vi "ANAL_TimeSummer.vi"(9 "Target Set Points":i32[](array[numeric]), 10 "Software Gate":cluster{"Numeric":i32, "Numeric":i32}, 11 "Run Data Cluster":T2 {"Temperature B" scale=0.0..100.0; "Temperature A" scale=0.0..100.0}) -> (2 "Time Array":T1(array[cluster]))   [LabVIEW 2021]
uses:
  DAT_Cluster.ctl
  2ce880be-73f0-4406-b417-1ac9331a85e2.vi
  2ce880be-73f0-4406-b417-1ac9331a85e2.vi/d4db2432-cc9c-482c-8957-dac855435ef6.vi
  2ce880be-73f0-4406-b417-1ac9331a85e2.vi/86fbf154-bd7b-49a2-8ab2-a837b2a95f24.vi
  2ce880be-73f0-4406-b417-1ac9331a85e2.vi/3b95b01e-1ec2-4565-bcd9-7606a5281010.vi
  2ce880be-73f0-4406-b417-1ac9331a85e2.vi/96a08935-737a-44b2-979c-a81d56408f7e.vi
  2ce880be-73f0-4406-b417-1ac9331a85e2.vi/d4db2432-cc9c-482c-8957-dac855435ef6.vi/6eaecd13-6e48-4772-a921-b51ebdf84d88.vi
  2ce880be-73f0-4406-b417-1ac9331a85e2.vi/d4db2432-cc9c-482c-8957-dac855435ef6.vi/d2d5f2b7-06f4-47f6-971c-049c3fdbb653.vi
  2ce880be-73f0-4406-b417-1ac9331a85e2.vi/3b95b01e-1ec2-4565-bcd9-7606a5281010.vi/6eaecd13-6e48-4772-a921-b51ebdf84d88.vi
  2ce880be-73f0-4406-b417-1ac9331a85e2.vi/3b95b01e-1ec2-4565-bcd9-7606a5281010.vi/d2d5f2b7-06f4-47f6-971c-049c3fdbb653.vi
  2ce880be-73f0-4406-b417-1ac9331a85e2.vi/96a08935-737a-44b2-979c-a81d56408f7e.vi/6eaecd13-6e48-4772-a921-b51ebdf84d88.vi
  2ce880be-73f0-4406-b417-1ac9331a85e2.vi/96a08935-737a-44b2-979c-a81d56408f7e.vi/d2d5f2b7-06f4-47f6-971c-049c3fdbb653.vi
  <vilib>/Comparison/Less/Less Functor/Less Functor.lvclass
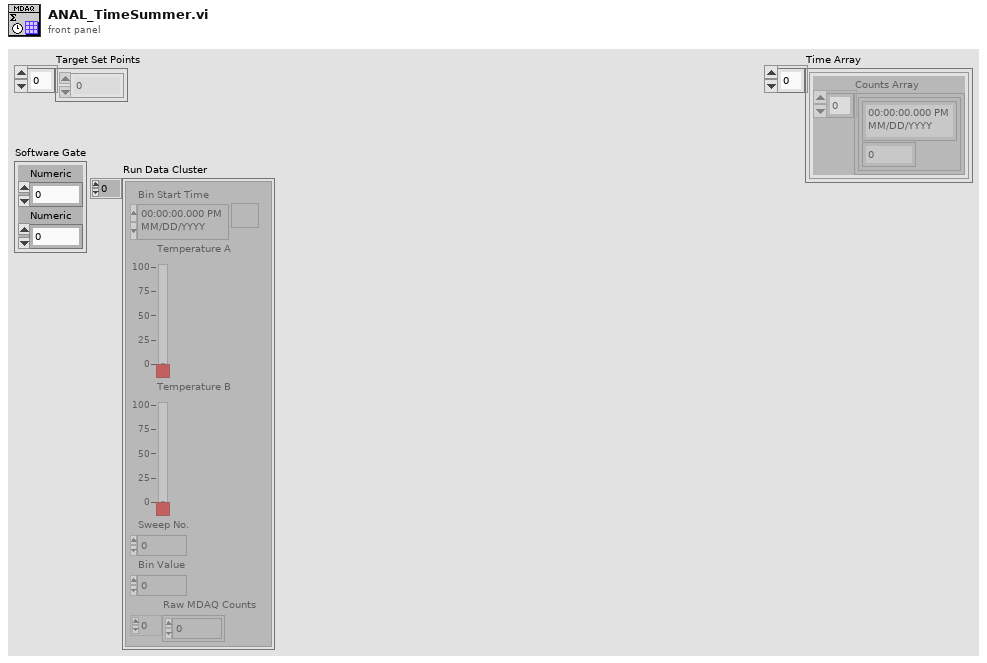
[diagram p1: front panel]
types:
  T1 = cluster{"Counts Array":cluster{timestamp, dbl}[]}[]
  T2 = typedef "DAT_Cluster.ctl" = cluster{"Bin Start Time":timestamp, "Temperature A":dbl, "Temperature B":dbl, "Sweep No.":i32, "Bin Value":i32, "Raw MDAQ Counts":i32[]}[]
  T3 = cluster{"Bin Start Time":timestamp, "Numeric":i32, "nearest index":i32}[]
  T4 = cluster{"Counts Array":cluster{timestamp, dbl}[]}
  T5 = cluster{"Bin Start Time":timestamp, "Numeric":i32, "nearest index":i32}
  T6 = cluster{"Bin Start Time":timestamp, "Numeric":i32}
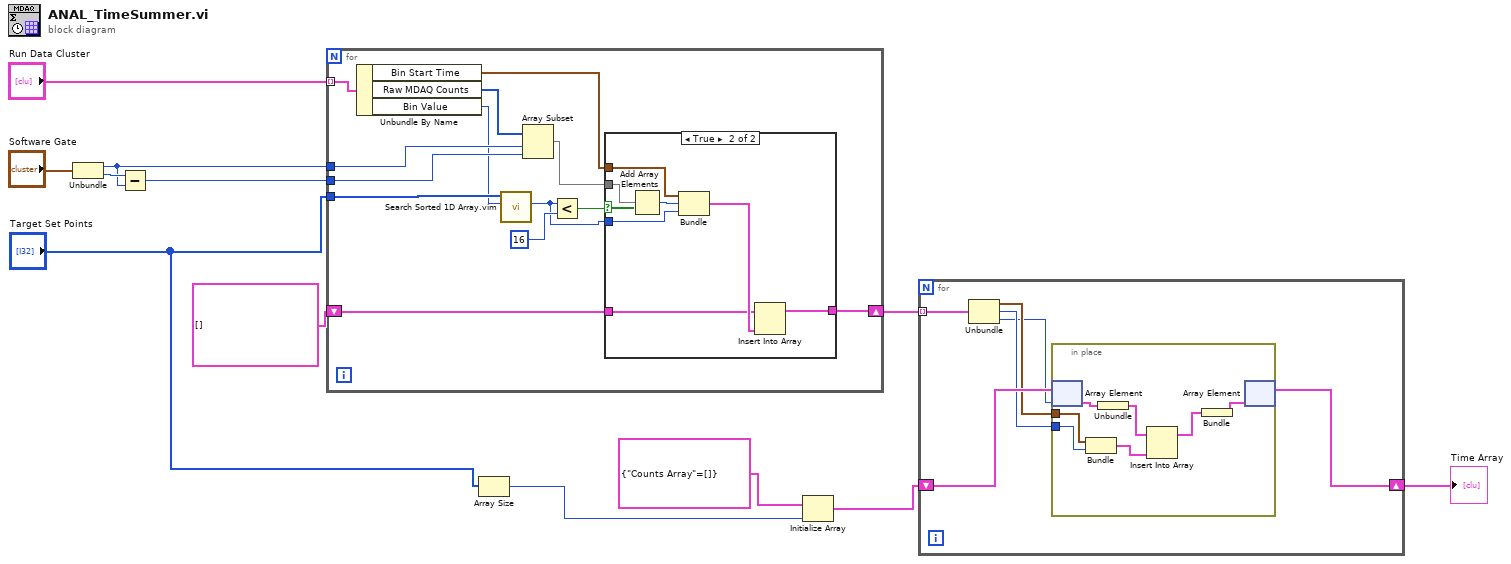
[diagram p0: block diagram]
diagram:
  n1 = Unbundle("Software Gate") -> ("Numeric"=w9:i32, "Numeric"=w10:i32)
  n2 = Subtract(x=w10, y=w9) -> (x-y=w8:i32)
  n3 = for {
    tunnel: "Run Data Cluster" -> [w25] mode=indexing
    tunnel: w9 -> [w23]
    tunnel: w8 -> [w22]
    tunnel: "Target Set Points" -> [w21]
    shift-right: [w14] -> w7
    shift-left: T3 [] ("array") -> [w15]
    n4 = Unbundle By Name(w25) -> ("Bin Start Time"=w18:timestamp, "Raw MDAQ Counts"=w24:i32[], "Bin Value"=w16:i32)
    n5 = call "Search Sorted 1D Array.vim"("element"=w16, "sorted 1D array"=w21) -> ("nearest index"=w13:i32)  [unwired: 8 in, 1 out]
    n6 = Array Subset(array=w24, index=w23, length=w22) -> (w17:i32[])
    n7 = Less?(x=w13, y=16) -> (x < y?=w19:bool)
    n8 = case shown="True" w19 {
      tunnel: w18 -> [_ w33]
      tunnel: w17 -> [_ w32]
      tunnel: w15 -> [w26 w27]
      tunnel: [w26 w28] -> w14
      tunnel: w13 -> [_ w30]
      frame False {
      }
      frame True {
        n9 = Add Array Elements(numeric array=w32) -> (sum=w31:i32)
        n10 = Bundle("Bin Start Time"=w33, "Numeric"=w31, "nearest index"=w30) -> (w29:T5)  [unwired: 1 in]
        n11 = Insert Into Array(array=w27, new element=w29) -> (w28:T3)  [unwired: 1 in]
      }
    }
  }
  n12 = Array Size(array="Target Set Points") -> (size(s)=w4:i32)
  n13 = Initialize Array(T4 {"Counts Array"=[]} ("Spectrum Array"), w4) -> (w3:T1)
  n14 = for {
    tunnel: w7 -> [w39] mode=indexing
    shift-right: [w37] -> w2
    shift-left: w3 -> [w38]
    n15 = Unbundle(w39) -> ("Bin Start Time"=w36:timestamp, "Numeric"=w35:i32, "nearest index"=w34:i32)
    n16 = in-place {
      in-place-border: w36 -> [w46]
      in-place-border: w35 -> [w45]
      n17 = in-place-array #1(w38, w34) -> (w44:T4)
      n18 = Bundle("Bin Start Time"=w46, "Numeric"=w45) -> (w42:T6)  [unwired: 1 in]
      n19 = Unbundle(w44) -> ("Counts Array"=w43:cluster{timestamp, dbl}[])
      n20 = Insert Into Array(array=w43, new element=w42) -> (w40:cluster{timestamp, dbl}[])  [unwired: 1 in]
      n21 = Bundle("Counts Array"=w40) -> (w41:T4)  [unwired: 1 in]
      n22 = in-place-array #1(w41) -> (w37:T1)  [unwired: 1 out]
    }
  }
  "Time Array" <- w2
